vi "Remote Unused References.vi"(8 "error in (no error)":errorcluster, 11 "Instrument.Lockin in":refnum<class "Instrument.Lockin.lvclass">) -> (0 "error out":errorcluster, 2 "Array":T1[](array[typedef]) {"References" items=["", "1", "2", "3"]}, 3 "Instrument.Lockin out":refnum<class "Instrument.Lockin.lvclass">)   [LabVIEW 2016, in "Instrument.Lockin.lvclass"]
uses:
  Instrument.Lockin.lvclass
  Instrument.Lockinl.UI/Typedefs/AI Channel--Cluster.ctl
  Instrument.Lockin.lvclass/Instrument.Lockin.ctl
  <userlib>/_OpenG.lib/array/array.llb/Delete Elements from 1D Array (U16)__ogtk.vi
  Instrument.Lockinl.UI/Instrument.Lockin.UI.lvclass
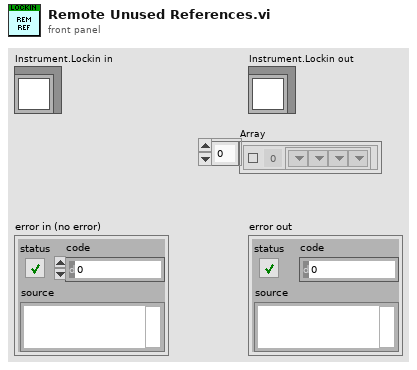
[diagram p1: front panel]
types:
  T1 = typedef "Instrument.Lockin.UI.lvclass/AI Channel--Cluster.ctl" = cluster{"Enable?":bool, "Channel":i32, "References":u16[]}
  T2 = typedef "Lockin.DAQ.lvclass/AI-cluster.ctl" = T1[]
  T3 = typedef "Lockin.DAQ.lvclass/REF-cluster.ctl" = T4[]
  T4 = typedef "Instrument.Lockin.UI.lvclass/REF Channel--Cluster.ctl" = cluster{"Enable?":bool, "Channel":i32, "Frequency":dbl, "Phase":dbl, "TC":dbl, "Order":i32}
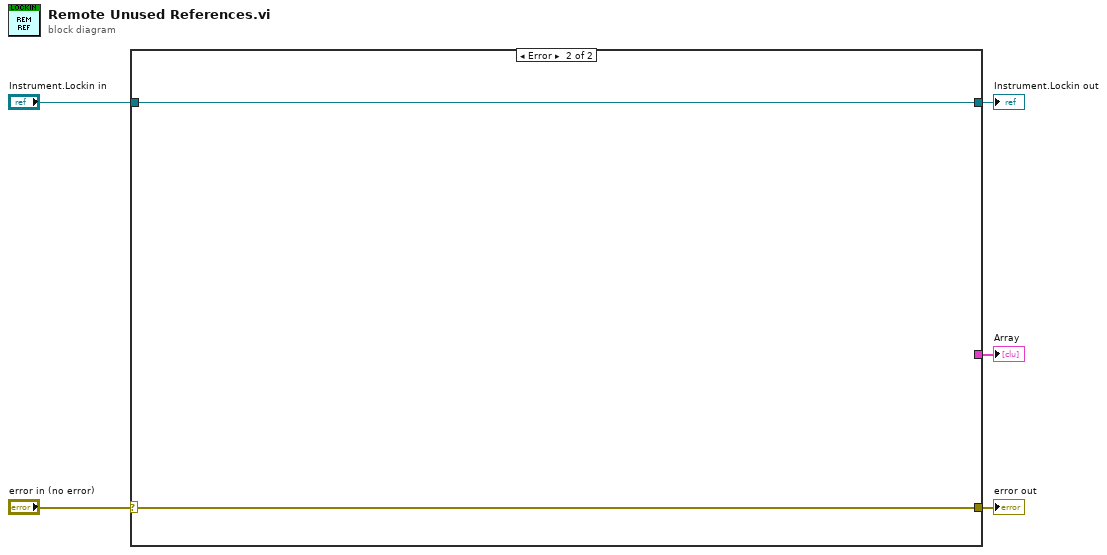
[diagram p0: block diagram]
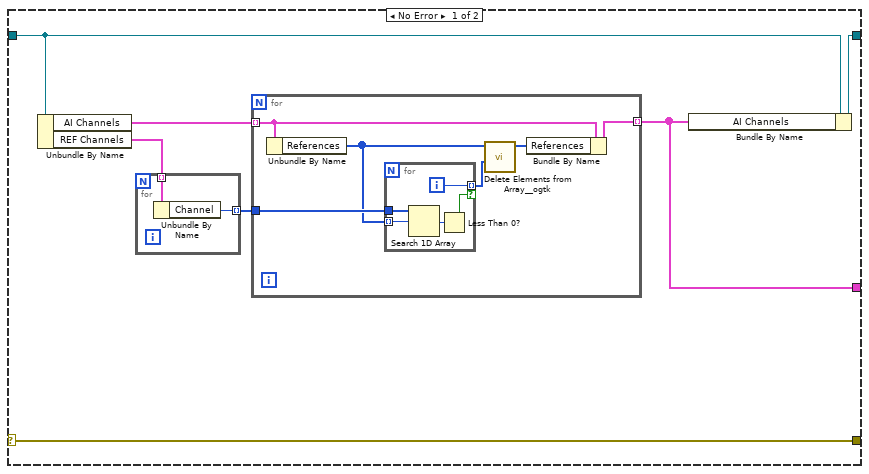
[diagram p2: hidden frame]
diagram:
  n1 = case shown="Error" "error in (no error)" {
    selector: "error in (no error)" -> [w6 w27]
    tunnel: [w12 w26] -> w5
    tunnel: "Instrument.Lockin in" -> [w11 w26]
    tunnel: [w7 _] -> w3
    tunnel: [w6 w27] -> w1
    frame No Error {
      n2 = Unbundle By Name(w11) -> ("AI Channels"=w10:T2, "REF Channels"=w8:T3)
      n3 = for {
        tunnel: [w14] -> w9 mode=indexing
        tunnel: w8 -> [w13] mode=indexing
        n4 = Unbundle By Name(w13) -> ("Channel"=w14:i32)
      }
      n5 = for {
        tunnel: w10 -> [w16] mode=indexing
        tunnel: w9 -> [w20]
        tunnel: [w17] -> w7 mode=indexing
        n6 = Unbundle By Name(w16) -> ("References"=w18:u16[])
        n7 = for {
          tunnel: w20 -> [w25]
          tunnel: w18 -> [w24] mode=indexing
          tunnel: [w22] -> w19 mode=indexing if=w21
          i -> [w22]
          n8 = Search 1D Array(1D array=w25, element=w24) -> (index of element=w23:i32)  [unwired: 1 in]
          n9 = Less Than 0?(x=w23) -> (x < 0?=w21:bool)
        }
        n10 = call-poly <userlib>:"Delete Elements from Array__ogtk.vi"("indices"=w19, "array"=w18) -> ("array w/ subset deleted"=w15:u16[])  [unwired: 8 in, 1 out]
        n11 = Bundle By Name(cluster=w16, "References"=w15) -> (w17:T1)
      }
      n12 = Bundle By Name(cluster=w11, "AI Channels"=w7) -> (w12:refnum<class "Instrument.Lockin.lvclass">)
    }
    frame Error {
    }
  }
  "error out" <- w1
  "Instrument.Lockin out" <- w5
  "Array" <- w3
